vi "Unit Set by item.vi"(9 "교정기능 2 리스트":string[](array[string]), 11 "분류코드":string) -> (0 "컬럼 헤더+CMC":string[](array[string]), 1 "컬럼 헤더":string[](array[string]), 2 "교정기능 2 리스트 2":string[](array[string]), 3 "교정기능 2 캡션":string, 4 "Condition2 캡션":string, 5 "콤보박스":T2, 6 "SQL query":string, 7 "클러스터":T1)   [LabVIEW 2020]
uses:
  Variables/Global_Constant.vi
  Public/Polymorph/Rmv Empt Arr_1D Str.vi
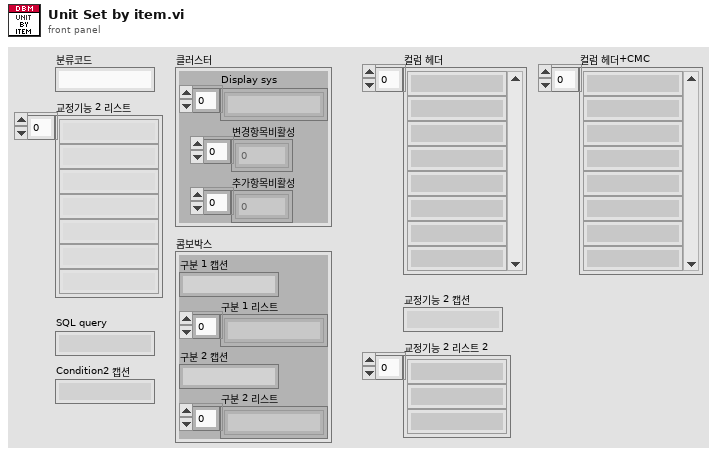
[diagram p1: front panel]
types:
  T1 = cluster{"Display sys":string[], "변경항목비활성":i32[], "추가항목비활성":i32[]}
  T2 = cluster{"구분 1 캡션":string, "구분 1 리스트":string[], "구분 2 캡션":string, "구분 2 리스트":string[]}
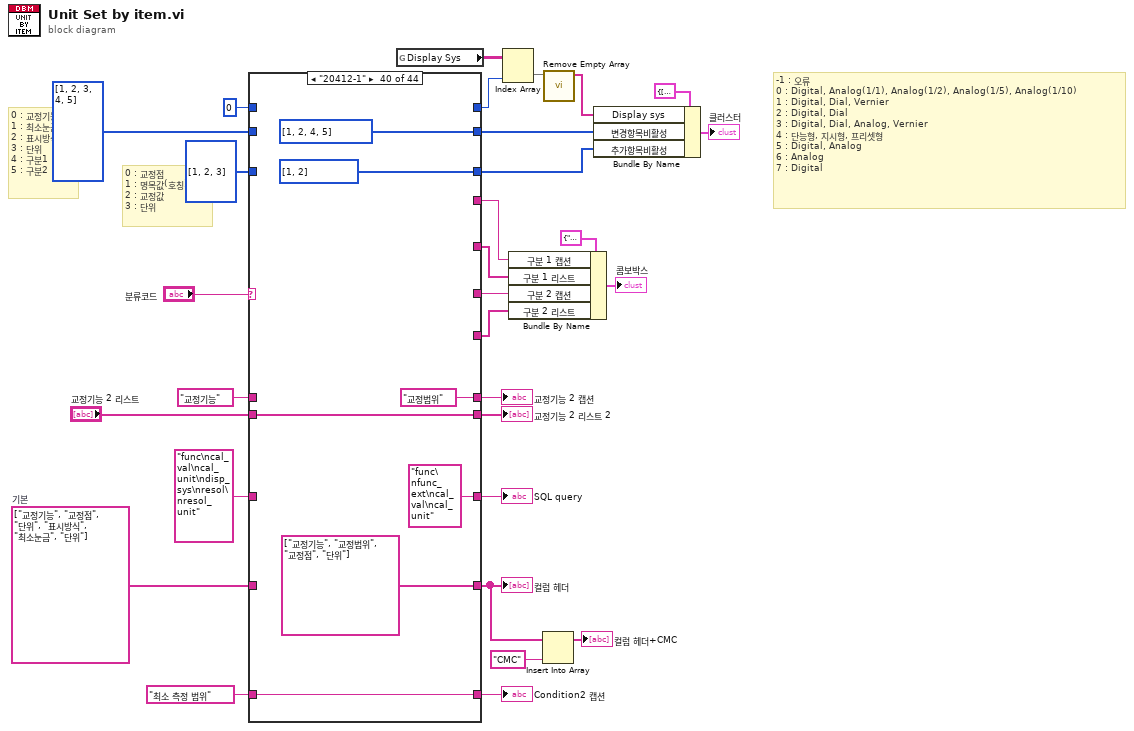
[diagram p0: block diagram]
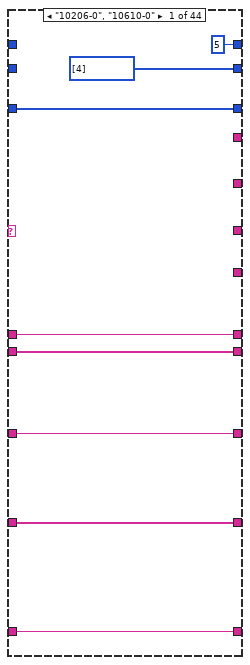
[diagram p2: hidden frame]
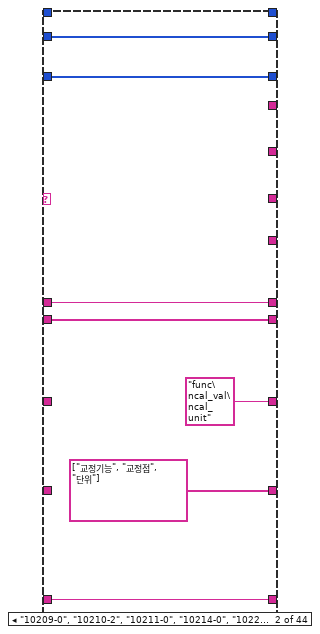
[diagram p3: hidden frame]
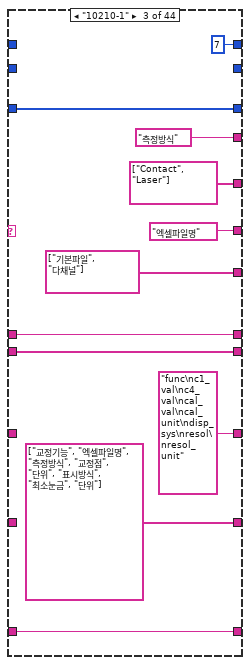
[diagram p4: hidden frame]
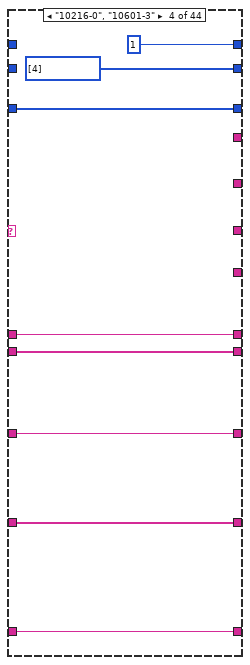
[diagram p5: hidden frame]
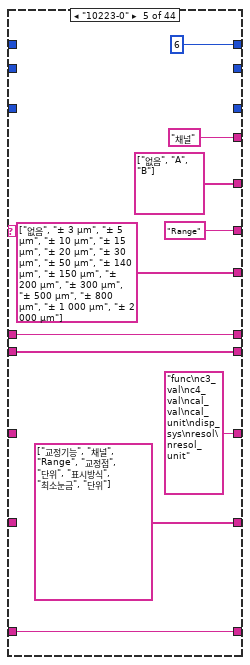
[diagram p6: hidden frame]
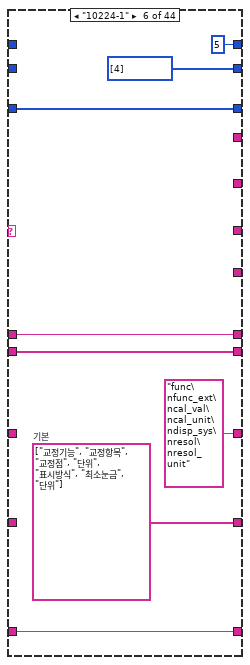
[diagram p7: hidden frame]
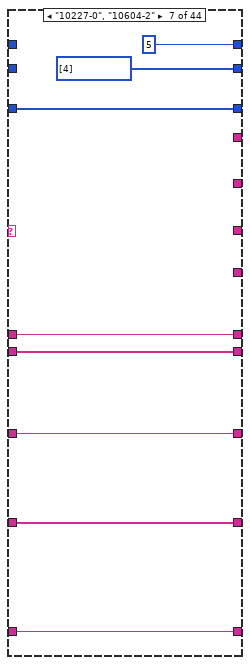
[diagram p8: hidden frame]
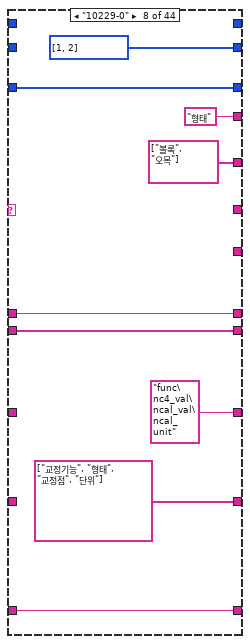
[diagram p9: hidden frame]
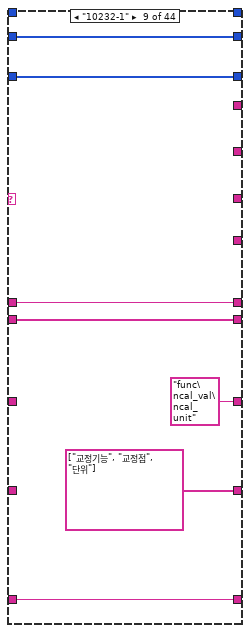
[diagram p10: hidden frame]
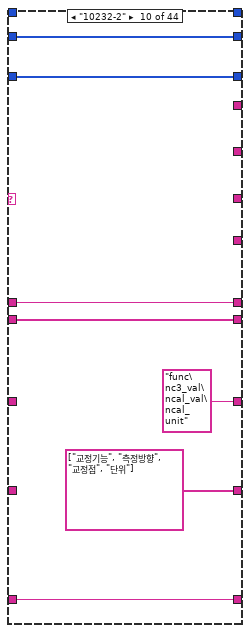
[diagram p11: hidden frame]
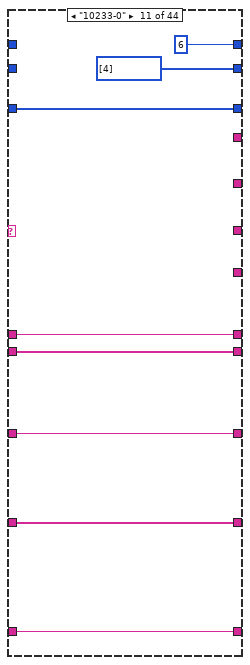
[diagram p12: hidden frame]
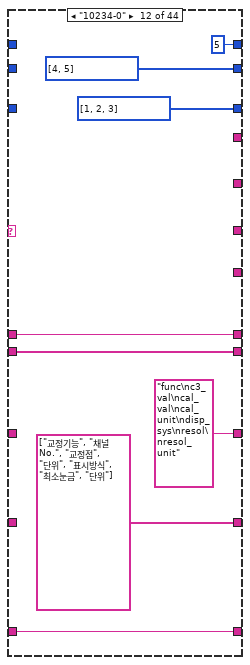
[diagram p13: hidden frame]
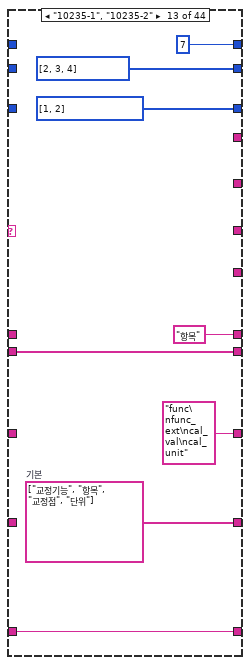
[diagram p14: hidden frame]
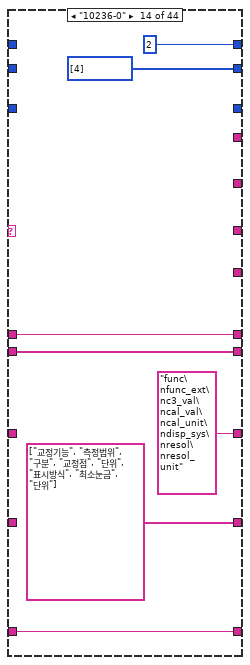
[diagram p15: hidden frame]
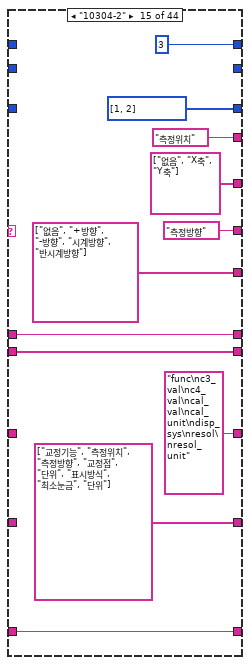
[diagram p16: hidden frame]
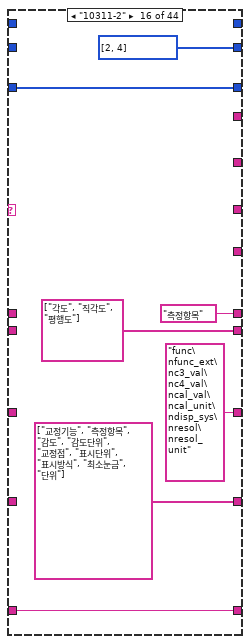
[diagram p17: hidden frame]
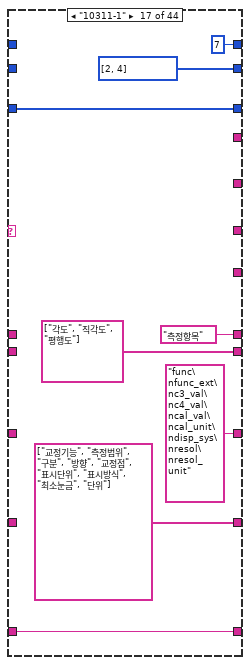
[diagram p18: hidden frame]
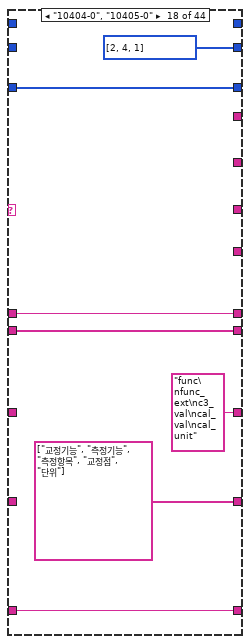
[diagram p19: hidden frame]
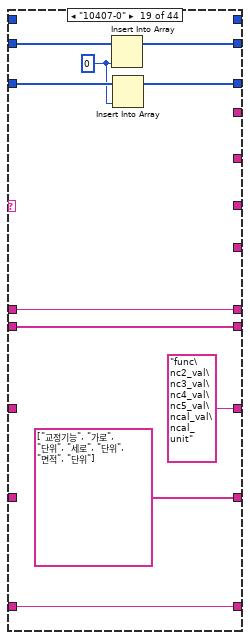
[diagram p20: hidden frame]
diagram:
  w26 = string[] ["교정기능", "교정점", "단위", "표시방식", "최소눈금", "단위"]  # 기본
  # "0 : 교정점\n1 : 명목값(호칭)\n2 : 교정값\n3 : 단위"
  # "0 : 교정기능\n1 : 최소눈금\n2 : 표시방식\n3 : 단위\n4 : 구분1\n5 : 구분2"
  # "-1 : 오류\n0 : Digital, Analog(1/1), Analog(1/2), Analog(1/5), Analog(1/10)\n1 : Digital, Dial, Vernier\n2 : Digital, Dial\n3 : Digital, Dial, Analog, Vernier\n4 : 단능형, 지시형, 프리셋형\n5 : Digital, Analog\n6 : Analog\n7 : Digital"
  n1 = case shown="\"20412-1\"" "분류코드" {
    tunnel: [w35 "func\ncal_val\ncal_unit" ("SQL query") "func\nc1_val\nc4_val\ncal_val\ncal_unit\ndisp_sys\nresol\nresol_unit" ("SQL query") w60 "func\nc3_val\nc4_val\ncal_val\ncal_unit\ndisp_sys\nresol\nresol_unit" ("SQL query") "func\nfunc_ext\ncal_val\ncal_unit\ndisp_sys\nresol\nresol_unit" ("SQL query") w87 "func\nc4_val\ncal_val\ncal_unit" ("SQL query") "func\ncal_val\ncal_unit" ("SQL query") "func\nc3_val\ncal_val\ncal_unit" ("SQL query") w119 "func\nc3_val\ncal_val\ncal_unit\ndisp_sys\nresol\nresol_unit" ("SQL query") "func\nfunc_ext\ncal_val\ncal_unit" ("SQL query") "func\nfunc_ext\nc3_val\ncal_val\ncal_unit\ndisp_sys\nresol\nresol_unit" ("SQL query") "func\nc3_val\nc4_val\ncal_val\ncal_unit\ndisp_sys\nresol\nresol_unit" ("SQL query") "func\nfunc_ext\nc3_val\nc4_val\ncal_val\ncal_unit\ndisp_sys\nresol\nresol_unit" ("SQL query") "func\nfunc_ext\nc3_val\nc4_val\ncal_val\ncal_unit\ndisp_sys\nresol\nresol_unit" ("SQL query") "func\nfunc_ext\nc3_val\ncal_val\ncal_unit" ("SQL query") "func\nc2_val\nc3_val\nc4_val\nc5_val\ncal_val\ncal_unit" ("SQL query") w189 "func\nfunc_ext\ncal_val\ncal_unit\ndisp_sys\nresol\nresol_unit" ("SQL query") "func\nfunc_ext\nc3_val\nc4_val\nc5_val\ncal_val\ncal_unit\ndisp_sys\nresol\nresol_unit" ("SQL query") "func\nfunc_ext\nc3_val\ncal_val\ncal_unit\ndisp_sys\nresol\nresol_unit" ("SQL query") w221 "func\nfunc_ext\nc3_val\ncal_val\ncal_unit\ndisp_sys\nresol\nresol_unit" ("SQL query") "func\nc3_val\ncal_val\ncal_unit\ndisp_sys\nresol\nresol_unit" ("SQL query") w247 "func\nc3_val\ncal_val\ncal_unit\ndisp_sys\nresol\nresol_unit" ("SQL query") w262 w274 "func\nfunc_ext\ncal_val\ncal_unit\nresol\nresol_unit" ("SQL query") "func\nfunc_ext\nc2_val\ncal_val\ncal_unit" ("SQL query") "func\nfunc_ext\nc2_val\nc3_val\nc4_val\nc5_val\ncal_val\ncal_unit" ("SQL query") "func\nfunc_ext\nc3_val\nc4_val\ncal_val\ncal_unit\ndisp_sys\nresol" ("SQL query") "func\nfunc_ext\nc3_val\ncal_val\ncal_unit\ndisp_sys\nresol\nresol_unit" ("SQL query") w320 w328 "func\nfunc_ext\ncal_val\ncal_unit\ndisp_sys\nresol\nresol_unit" ("SQL query") "func\nfunc_ext\nc4_val\ncal_unit\ndisp_sys\nresol\nresol_unit" ("SQL query") "func\nfunc_ext\ncal_val\ncal_unit" ("SQL query") "func\nfunc_ext\ncal_val\ncal_unit" ("SQL query") "func\nfunc_ext\ncal_val\ncal_unit" ("SQL query") "func\nfunc_ext\nc3_val\nc4_val\ncal_val\ncal_unit\ndisp_sys\nresol\nresol_unit" ("SQL query") w383] -> w25
    tunnel: [w36 string[] ["교정기능", "교정점", "단위"] ("문자열[]") string[] ["교정기능", "엑셀파일명", "측정방식", "교정점", "단위", "표시방식", "최소눈금", "단위"] w62 string[] ["교정기능", "채널", "Range", "교정점", "단위", "표시방식", "최소눈금", "단위"] ("문자열[]") w77 w89 string[] ["교정기능", "형태", "교정점", "단위"] ("문자열[]") string[] ["교정기능", "교정점", "단위"] ("기본") string[] ["교정기능", "측정방향", "교정점", "단위"] ("기본") w118 string[] ["교정기능", "채널 No.", "교정점", "단위", "표시방식", "최소눈금", "단위"] ("기본") w133 string[] ["교정기능", "측정범위", "구분", "교정점", "단위", "표시방식", "최소눈금", "단위"] ("문자열[]") string[] ["교정기능", "측정위치", "측정방향", "교정점", "단위", "표시방식", "최소눈금", "단위"] ("문자열[]") string[] ["교정기능", "측정항목", "감도", "감도단위", "교정점", "표시단위", "표시방식", "최소눈금", "단위"] ("문자열[]") string[] ["교정기능", "측정범위", "구분", "방향", "교정점", "표시단위", "표시방식", "최소눈금", "단위"] ("문자열[]") string[] ["교정기능", "측정기능", "측정항목", "교정점", "단위"] ("문자열[]") string[] ["교정기능", "가로", "단위", "세로", "단위", "면적", "단위"] ("문자열[]") w188 string[] ["교정기능", "세부기능", "교정점", "단위", "표시방식", "최소눈금", "단위"] string[] ["교정기능", "세부기능", "측정방향", "측정구간", "단위", "교정점", "단위", "표시방식", "최소눈금", "단위"] string[] ["교정기능", "측정범위", "배율", "교정점", "단위", "표시방식", "최소눈금", "단위"] ("문자열[]") w220 w229 string[] ["교정기능", "측정위치", "교정점", "단위", "표시방식", "최소눈금", "단위"] ("문자열[]") w249 string[] ["교정기능", "측정방향", "교정점", "단위", "표시방식", "최소눈금", "단위"] ("문자열[]") w263 w276 w285 w293 w301 string[] ["교정기능", "세부기능", "최대지시값", "지시단위", "교정점", "단위", "표시방식", "최소눈금"] ("문자열[]") string[] ["교정기능", "세부기능", "구분", "교정점", "단위", "표시방식", "최소눈금", "단위"] ("문자열[]") w321 w329 w338 w346 string[] ["교정기능", "교정범위", "교정점", "단위"] string[] ["교정기능", "교정범위", "교정점", "단위"] string[] ["교정기능", "교정범위", "교정점", "단위"] w376 w384] -> w4
    tunnel: [w37 w43 w52 w63 w71 w81 w90 w97 w105 w112 w117 w125 "항목" ("캡션.텍스트") w141 w152 "측정항목" ("캡션.텍스트") "측정항목" ("캡션.텍스트") w172 w184 w192 "세부기능" ("캡션.텍스트") "세부기능" ("캡션.텍스트") w216 w223 w232 "측정위치" ("캡션.텍스트") w250 w257 w268 w277 "측정범위" ("캡션.텍스트") "교정품목" ("캡션.텍스트") "교정품목" ("캡션.텍스트") w307 w316 w325 w333 "교정범위" ("캡션.텍스트") "교정범위" ("캡션.텍스트") "교정범위" ("캡션.텍스트") "교정범위" ("캡션.텍스트") "교정범위" ("캡션.텍스트") "교정범위" ("캡션.텍스트") w385] -> w12
    tunnel: [w38 w42 w53 w61 w70 w82 w88 w96 w104 w111 w116 w124 w135 w140 w151 string[] ["각도", "직각도", "평행도"] ("교정기능 문자열[]") string[] ["각도", "직각도", "평행도"] ("교정기능 문자열[]") w173 w185 w193 w202 w210 w215 w222 w231 string[] ["Outside", "Inside"] ("문자열[]") w248 w256 w267 w275 w282 w290 w298 w306 w315 w324 w332 w336 w344 w352 w359 w366 w374 w386] -> w11
    tunnel: "교정기능 2 리스트" -> [w38 w42 w53 w61 w70 w82 w88 w96 w104 w111 w116 w124 w135 w140 w151 _ _ w173 w185 w193 w202 w210 w215 w222 w231 _ w248 w256 w267 w275 w282 w290 w298 w306 w315 w324 w332 w336 w344 w352 w359 w366 w374 w386]
    tunnel: "교정기능" ("캡션.텍스트") -> [w37 w43 w52 w63 w71 w81 w90 w97 w105 w112 w117 w125 _ w141 w152 _ _ w172 w184 w192 _ _ w216 w223 w232 _ w250 w257 w268 w277 _ _ _ w307 w316 w325 w333 _ _ _ _ _ _ w385]
    tunnel: w26 -> [w36 _ _ w62 _ _ w89 _ _ _ w118 _ _ _ _ _ _ _ _ w188 _ _ _ w220 _ _ w249 _ w263 w276 _ _ _ _ _ w321 w329 _ _ _ _ _ _ w384]
    tunnel: "func\ncal_val\ncal_unit\ndisp_sys\nresol\nresol_unit" ("SQL query") -> [w35 _ _ w60 _ _ w87 _ _ _ w119 _ _ _ _ _ _ _ _ w189 _ _ _ w221 _ _ w247 _ w262 w274 _ _ _ _ _ w320 w328 _ _ _ _ _ _ w383]
    tunnel: [5 ("비활성화된 인덱스 (열)") _ 7 ("비활성화된 인덱스 (열)") 1 ("비활성화된 인덱스 (열)") 6 ("비활성화된 인덱스 (열)") 5 ("비활성화된 인덱스 (열)") 5 ("비활성화된 인덱스 (열)") _ _ _ 6 ("비활성화된 인덱스 (열)") 5 ("비활성화된 인덱스 (열)") 7 ("비활성화된 인덱스 (열)") 2 ("비활성화된 인덱스 (열)") 3 ("비활성화된 인덱스 (열)") _ 7 ("비활성화된 인덱스 (열)") _ _ 6 ("비활성화된 인덱스 (열)") 7 ("비활성화된 인덱스 (열)") 7 ("비활성화된 인덱스 (열)") 7 ("비활성화된 인덱스 (열)") w225 7 ("비활성화된 인덱스 (열)") 1 ("비활성화된 인덱스 (열)") 2 ("비활성화된 인덱스 (열)") 2 ("비활성화된 인덱스 (열)") 5 ("비활성화된 인덱스 (열)") 8 ("비활성화된 인덱스 (열)") w279 w287 w295 _ w309 1 ("비활성화된 인덱스 (열)") 4 ("비활성화된 인덱스 (열)") 0 ("비활성화된 인덱스 (열)") 0 ("비활성화된 인덱스 (열)") _ _ _ w372 w380] -> w8
    tunnel: [i32[] [4] w40 _ i32[] [4] _ i32[] [4] i32[] [4] i32[] [1, 2] w101 w108 i32[] [4] i32[] [4, 5] i32[] [2, 3, 4] i32[] [4] _ i32[] [2, 4] i32[] [2, 4] i32[] [2, 4, 1] w181 i32[] [4, 5, 3] i32[] [4, 5] i32[] [4, 5] i32[] [4, 5] i32[] [4, 5] i32[] [4, 5] i32[] [4] i32[] [4] i32[] [4] i32[] [4] i32[] [4] i32[] [2, 4] i32[] [0, 1, 2, 3, 4] i32[] [0, 1, 2, 3, 4] i32[] [4] _ i32[] [0] i32[] [0, 4] i32[] [4] i32[] [4] i32[] [1, 2, 4, 5] i32[] [1, 2, 4, 5] i32[] [1, 2, 4, 5] i32[] [2, 3, 4] i32[] [4]] -> w20
    tunnel: [w33 w41 w51 w58 _ w79 w84 w95 w100 w107 w115 i32[] [1, 2, 3] i32[] [1, 2] _ i32[] [1, 2] w159 w167 w174 w179 w194 w198 w206 w212 _ w227 w236 w244 w252 w264 w271 w280 i32[] [0] i32[] [0] w304 w313 w319 w327 i32[] [1, 2] i32[] [1, 2] i32[] [1, 2] i32[] [1, 2] i32[] [1, 2] i32[] [1, 2] w381] -> w19
    tunnel: i32[] [1, 2, 3] -> [w33 w41 w51 w58 _ w79 w84 w95 w100 w107 w115 _ _ _ _ w159 w167 w174 w180 w194 w198 w206 w212 _ w227 w236 w244 w252 w264 w271 w280 _ _ w304 w313 w319 w327 _ _ _ _ _ _ w381]
    tunnel: [_ _ "측정방식" _ "채널" _ _ "형태" _ _ _ _ _ _ "측정위치" _ _ _ _ _ _ _ _ _ _ _ _ "측정방향" "측정방향" _ _ _ _ _ "구분" _ _ _ _ _ _ _ _ _] -> w17
    tunnel: [_ _ string[] ["Contact", "Laser"] _ string[] ["없음", "A", "B"] _ _ string[] ["볼록", "오목"] _ _ _ _ _ _ string[] ["없음", "X축", "Y축"] _ _ _ _ _ _ _ _ _ _ _ _ string[] ["시계방향", "반시계방향"] _ _ _ _ _ _ string[] ["Push Pull Gauge", "Tension Gauge"] _ _ _ _ _ _ _ _ _] -> w16
    tunnel: [_ _ "엑셀파일명" _ "Range" _ _ _ _ _ _ _ _ _ "측정방향" _ _ _ _ _ _ _ _ _ _ _ _ _ _ _ _ _ _ _ _ _ _ _ _ _ _ _ _ _] -> w15
    tunnel: [_ _ string[] ["기본파일", "다채널"] _ string[] ["없음", "± 3 μm", "± 5 μm", "± 10 μm", "± 15 μm", "± 20 μm", "± 30 μm", "± 50 μm", "± 140 μm", "± 150 μm", "± 200 μm", "± 300 μm", "± 500 μm", "± 800 μm", "± 1 000 μm", "± 2 000 μm"] _ _ _ _ _ _ _ _ _ string[] ["없음", "+방향", "-방향", "시계방향", "반시계방향"] _ _ _ _ _ _ _ _ _ _ _ _ _ _ _ _ _ _ _ _ _ _ _ _ _ _ _ _ _] -> w14
    tunnel: i32[] [1, 2, 3, 4, 5] -> [_ w40 _ _ _ _ _ _ w101 w108 _ _ _ _ _ _ _ _ w182 _ _ _ _ _ _ _ _ _ _ _ _ _ _ _ _ _ _ _ _ _ _ _ _ _]
    tunnel: 0 -> [_ _ _ _ _ _ _ _ _ _ _ _ _ _ _ _ _ _ _ _ _ _ _ w225 _ _ _ _ _ _ w279 w287 w295 _ w309 _ _ _ _ _ _ _ w372 w380]
    tunnel: [w32 w39 w46 w57 w65 w76 w83 w91 w106 w113 w114 w129 w130 w138 w145 w156 w164 w171 w183 w191 w196 w204 "배율" w226 w234 w235 w243 w251 w261 w270 w278 w286 w294 w302 w310 w318 w326 w334 w342 w350 w357 w364 w371 w379] -> w2
    tunnel: "최소 측정 범위" -> [w32 w39 w46 w57 w65 w76 w83 w91 w106 w113 w114 w129 w130 w138 w145 w156 w164 w171 w183 w191 w196 w204 _ w226 w234 w235 w243 w251 w261 w270 w278 w286 w294 w302 w310 w318 w326 w334 w342 w350 w357 w364 w371 w379]
    frame "10206-0", "10610-0" {
    }
    frame "10209-0", "10210-2", "10211-0", "10214-0", "10228-2" {
    }
    frame "10210-1" {
    }
    frame "10216-0", "10601-3" {
    }
    frame "10223-0" {
    }
    frame "10224-1" {
      w77 = string[] ["교정기능", "교정항목", "교정점", "단위", "표시방식", "최소눈금", "단위"]  # 기본
    }
    frame "10227-0", "10604-2" {
    }
    frame "10229-0" {
    }
    frame "10232-1" {
    }
    frame "10232-2" {
    }
    frame "10233-0" {
    }
    frame "10234-0" {
    }
    frame "10235-1", "10235-2" {
      w133 = string[] ["교정기능", "항목", "교정점", "단위"]  # 기본
    }
    frame "10236-0" {
    }
    frame "10304-2" {
    }
    frame "10311-2" {
    }
    frame "10311-1" {
    }
    frame "10404-0", "10405-0" {
    }
    frame "10407-0" {
      w178 = 0 ("새 원소/부분배열")
      n2 = Insert Into Array(array=w182, new element=w178) -> (w181:i32[])  [unwired: 1 in]
      n3 = Insert Into Array(array=w180, new element=w178) -> (w179:i32[])  [unwired: 1 in]
    }
    frame "10413-0" {
    }
    frame "10504-1", "10511-1", "10511-2" {
    }
    frame "10503-0" {
    }
    frame "10511-3" {
    }
    frame "10512-0" {
    }
    frame "10517-0" {
      w229 = string[] ["교정기능", "세부교정기능", "교정항목", "교정점", "단위", "표시방식", "최소눈금", "단위"]  # 기본
    }
    frame "10601-1" {
    }
    frame "10603-1", "10603-2", "10604-1", "10605-1", "10605-2" {
    }
    frame "10609-1" {
    }
    frame "10612-1", "10612-2" {
    }
    frame "10613-1" {
    }
    frame "20109-0" {
      w285 = string[] ["교정기능", "측정범위", "교정점", "단위", "최소눈금", "단위"]  # 20109-0
    }
    frame "20116-1" {
      w293 = string[] ["교정기능", "교정품목", "명목값", "교정값", "단위"]  # 20116-1
    }
    frame "20116-2" {
      w301 = string[] ["교정기능", "교정품목", "호칭", "교정값", "단위", "환산값(g)", "교정값", "단위"]  # 20116-2
    }
    frame "20202-0" {
    }
    frame "20204-0" {
    }
    frame "20302-0" {
    }
    frame "20303-0" {
    }
    frame "20406-0", "20408-0", "20411-1", "20411-4", "20413-0" {
      w338 = string[] ["교정기능", "교정범위", "교정점", "단위", "표시방식", "최소눈금", "단위"]  # 20406-0
    }
    frame "20409-0" {
      w346 = string[] ["교정기능", "교정범위", "교정점", "단위", "표시방식", "최소눈금", "단위"]  # 20406-0
    }
    frame "20412-1" {
    }
    frame "20412-2" {
    }
    frame "20412-3" {
    }
    frame "20414-0" {
      w376 = string[] ["교정기능", "교정범위", "기준수심", "단위", "교정점", "단위", "표시방식", "최소눈금", "단위"]  # 20414-0
    }
    frame Default {
    }
  }
  "SQL query" <- w25
  "컬럼 헤더" <- w4
  "교정기능 2 캡션" <- w12
  "교정기능 2 리스트 2" <- w11
  "Condition2 캡션" <- w2
  n4 = global read "Global_Constant.vi" "Display Sys"() -> (w9:string[][])
  n5 = Index Array(array=w9, index (col)=w8) -> (element=w10:string[])  [unwired: 1 in]
  n6 = Bundle By Name(cluster=T2 {"구분 1 캡션"="", "구분 1 리스트"=[], "구분 2 캡션"="", "구분 2 리스트"=[]}, "구분 1 캡션"=w17, "구분 1 리스트"=w16, "구분 2 캡션"=w15, "구분 2 리스트"=w14) -> (→"콤보박스":T2)
  n7 = Insert Into Array(array=w4, new element="CMC") -> (→"컬럼 헤더+CMC":string[])  [unwired: 1 in]
  n8 = call-poly "Remove Empty Array.vi"("Data in"=w10) -> ("Data out"=w7:string[])  [unwired: 9 in, 1 out]
  n9 = Bundle By Name(cluster=T1 {"Display sys"=[], "변경항목비활성"=[], "추가항목비활성"=[]}, "Display sys"=w7, "변경항목비활성"=w20, "추가항목비활성"=w19) -> (→"클러스터":T1)
